vi "test Sort Array of Clusters Natural String Sort.vi"(8 "error in (no error)":errorcluster, 11 "TestCase in":refnum<class "UI Common Unit Tests.lvclass">) -> (0 "error out":errorcluster, 3 "TestCase out":refnum<class "UI Common Unit Tests.lvclass">)   [LabVIEW 2020, in "UI Common Unit Tests.lvclass"]
uses:
  UI Common Unit Tests.lvclass
  Array Row.ctl
  63dc8703-c824-4b80-a085-58f57073aca5.vi
  d8dc5a30-59fd-40f1-b092-92b0634dc405.vi
  c62d43f3-ccf2-448e-89d3-d67a32af4b30.vi
  0d07b81e-88f3-4258-8836-385d3b76f707.vi
  63dc8703-c824-4b80-a085-58f57073aca5.vi/17eb59a9-6c8d-4297-8837-a139101b69e3.vi
  63dc8703-c824-4b80-a085-58f57073aca5.vi/21fb22a7-51bf-438c-989a-8269563528b1.vi
  d8dc5a30-59fd-40f1-b092-92b0634dc405.vi/3dcb3647-a2db-4cc0-b8b0-9940c197a0ae.vi
  d8dc5a30-59fd-40f1-b092-92b0634dc405.vi/7ad83155-26e6-464b-9375-e5ccdfa048ad.vi
  c62d43f3-ccf2-448e-89d3-d67a32af4b30.vi/ff9fbd3b-addb-4ece-97e3-770648744281.vi
  c62d43f3-ccf2-448e-89d3-d67a32af4b30.vi/64bd4fbf-d20b-4850-a5e4-08fff181ae49.vi
  0d07b81e-88f3-4258-8836-385d3b76f707.vi/ee9bf504-fb10-4b90-8e22-e8104f991147.vi
  0d07b81e-88f3-4258-8836-385d3b76f707.vi/d559d978-f639-4814-b0fe-533ccc604d91.vi
  Natural String Merge Sort.vi
  <vilib>/addons/_JKI Toolkits/VI Tester/TestCase.llb/TestCase.lvclass
  C:/Program Files (x86)/National Instruments/LabVIEW 2020/vi.lib/addons/_JKI Toolkits/VI Tester/TestCase.llb/TestCase.lvclass
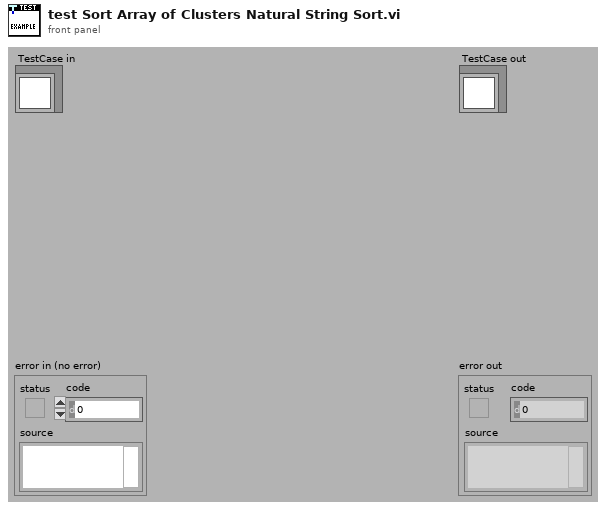
[diagram p1: front panel]
types:
  T1 = typedef "UI Common Unit Tests.lvclass/Array Row.ctl" = cluster{"String":string, "Numeric":dbl}
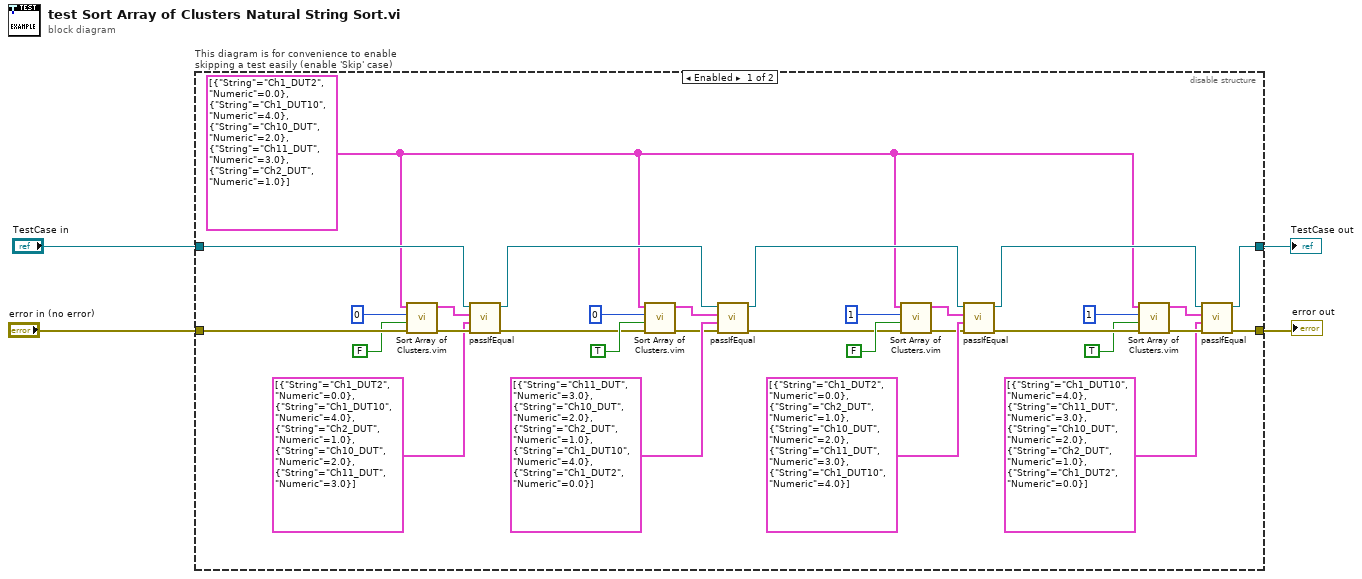
[diagram p0: block diagram]
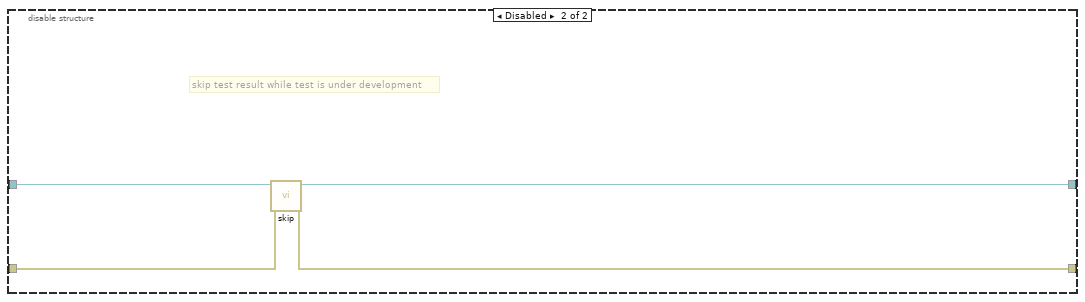
[diagram p2: hidden frame]
diagram:
  n1 = disable-structure "This diagram is for convenience to enable skipping a test easily (enable 'Skip' case)" shown="Enabled" {
    disable-tunnel: "TestCase in" -> [w31 w39]
    disable-tunnel: [w10 w37] -> w1
    disable-tunnel: [w6 w38] -> w3
    disable-tunnel: "error in (no error)" -> [w35 w36]
    frame Enabled {
      w5 = T1[] [{"String"="Ch1_DUT2", "Numeric"=0.0}, {"String"="Ch1_DUT10", "Numeric"=4.0}, {"String"="Ch10_DUT", "Numeric"=2.0}, {"String"="Ch11_DUT", "Numeric"=3.0}, {"String"="Ch2_DUT", "Numeric"=1.0}] ("Value")
      n2 = call "Sort Array of Clusters.vim"("error in (no error)"=w35, "Descending"=FALSE, "index"=u32 0, "Array"=w5) -> ("error out"=w32:errorcluster, "Sorted Array"=w30:T1[])  [unwired: 6 in]
      n3 = call-dynamic "passIfEqual.vi"("error in (no error)"=w32, "y"=T1[] [{"String"="Ch1_DUT2", "Numeric"=0.0}, {"String"="Ch1_DUT10", "Numeric"=4.0}, {"String"="Ch2_DUT", "Numeric"=1.0}, {"String"="Ch10_DUT", "Numeric"=2.0}, {"String"="Ch11_DUT", "Numeric"=3.0}] ("Value"), "x"=w30, "TestCase in"=w31) -> ("error out"=w23:errorcluster, "TestCase out"=w22:refnum<class "UI Common Unit Tests.lvclass">)  [unwired: 6 in]
      n4 = call "Sort Array of Clusters.vim"("error in (no error)"=w23, "Descending"=TRUE, "index"=u32 0, "Array"=w5) -> ("error out"=w26:errorcluster, "Sorted Array"=w27:T1[])  [unwired: 6 in]
      n5 = call-dynamic "passIfEqual.vi"("error in (no error)"=w26, "y"=T1[] [{"String"="Ch11_DUT", "Numeric"=3.0}, {"String"="Ch10_DUT", "Numeric"=2.0}, {"String"="Ch2_DUT", "Numeric"=1.0}, {"String"="Ch1_DUT10", "Numeric"=4.0}, {"String"="Ch1_DUT2", "Numeric"=0.0}] ("Value"), "x"=w27, "TestCase in"=w22) -> ("error out"=w7:errorcluster, "TestCase out"=w8:refnum<class "UI Common Unit Tests.lvclass">)  [unwired: 6 in]
      n6 = call "Sort Array of Clusters.vim"("error in (no error)"=w7, "Descending"=FALSE, "index"=u32 1, "Array"=w5) -> ("error out"=w13:errorcluster, "Sorted Array"=w14:T1[])  [unwired: 6 in]
      n7 = call-dynamic "passIfEqual.vi"("error in (no error)"=w13, "y"=T1[] [{"String"="Ch1_DUT2", "Numeric"=0.0}, {"String"="Ch2_DUT", "Numeric"=1.0}, {"String"="Ch10_DUT", "Numeric"=2.0}, {"String"="Ch11_DUT", "Numeric"=3.0}, {"String"="Ch1_DUT10", "Numeric"=4.0}] ("Value"), "x"=w14, "TestCase in"=w8) -> ("error out"=w21:errorcluster, "TestCase out"=w9:refnum<class "UI Common Unit Tests.lvclass">)  [unwired: 6 in]
      n8 = call "Sort Array of Clusters.vim"("error in (no error)"=w21, "Descending"=TRUE, "index"=u32 1, "Array"=w5) -> ("error out"=w18:errorcluster, "Sorted Array"=w17:T1[])  [unwired: 6 in]
      n9 = call-dynamic "passIfEqual.vi"("error in (no error)"=w18, "y"=T1[] [{"String"="Ch1_DUT10", "Numeric"=4.0}, {"String"="Ch11_DUT", "Numeric"=3.0}, {"String"="Ch10_DUT", "Numeric"=2.0}, {"String"="Ch2_DUT", "Numeric"=1.0}, {"String"="Ch1_DUT2", "Numeric"=0.0}] ("Value"), "x"=w17, "TestCase in"=w9) -> ("error out"=w6:errorcluster, "TestCase out"=w10:refnum<class "UI Common Unit Tests.lvclass">)  [unwired: 6 in]
    }
    frame Disabled {
      # "skip test result while test is under development"
      n10 = call <vilib>:"skip.vi"("error in (no error)"=w36, "TestCase in"=w39) -> ("error out"=w38:errorcluster, "TestCase out"=w37:refnum<class "UI Common Unit Tests.lvclass">)  [unwired: 8 in]
    }
  }
  "error out" <- w3
  "TestCase out" <- w1
